vi "Timing FGV.vi"(5 "Time Target (s)":i32=4, 7 "Timer Mode":T1(ring), 8 "Error In":errorcluster) -> (0 "Error Out":errorcluster, 2 "Elapsed Time (s.ms)":dbl format="%#.2f", 3 "Has Time Elapsed":bool)   [LabVIEW 2025, in "Config Tool.lvlib"]
doc: "CLD 3 Exercise\nThis VI is used as a timer functional global. \nNote on reading time when in pause. The developer should not call the read time function when in pause; however, a case structure is used to defensively program the read state for this possibility."
uses:
  Config Tool.lvlib
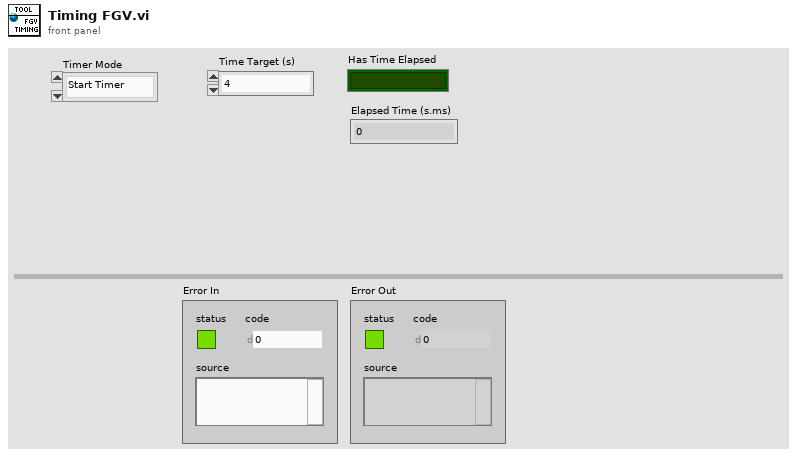
[diagram p1: front panel]
types:
  T1 = enum16{"Start Timer", "Read Time", "Pause", "Resume"}
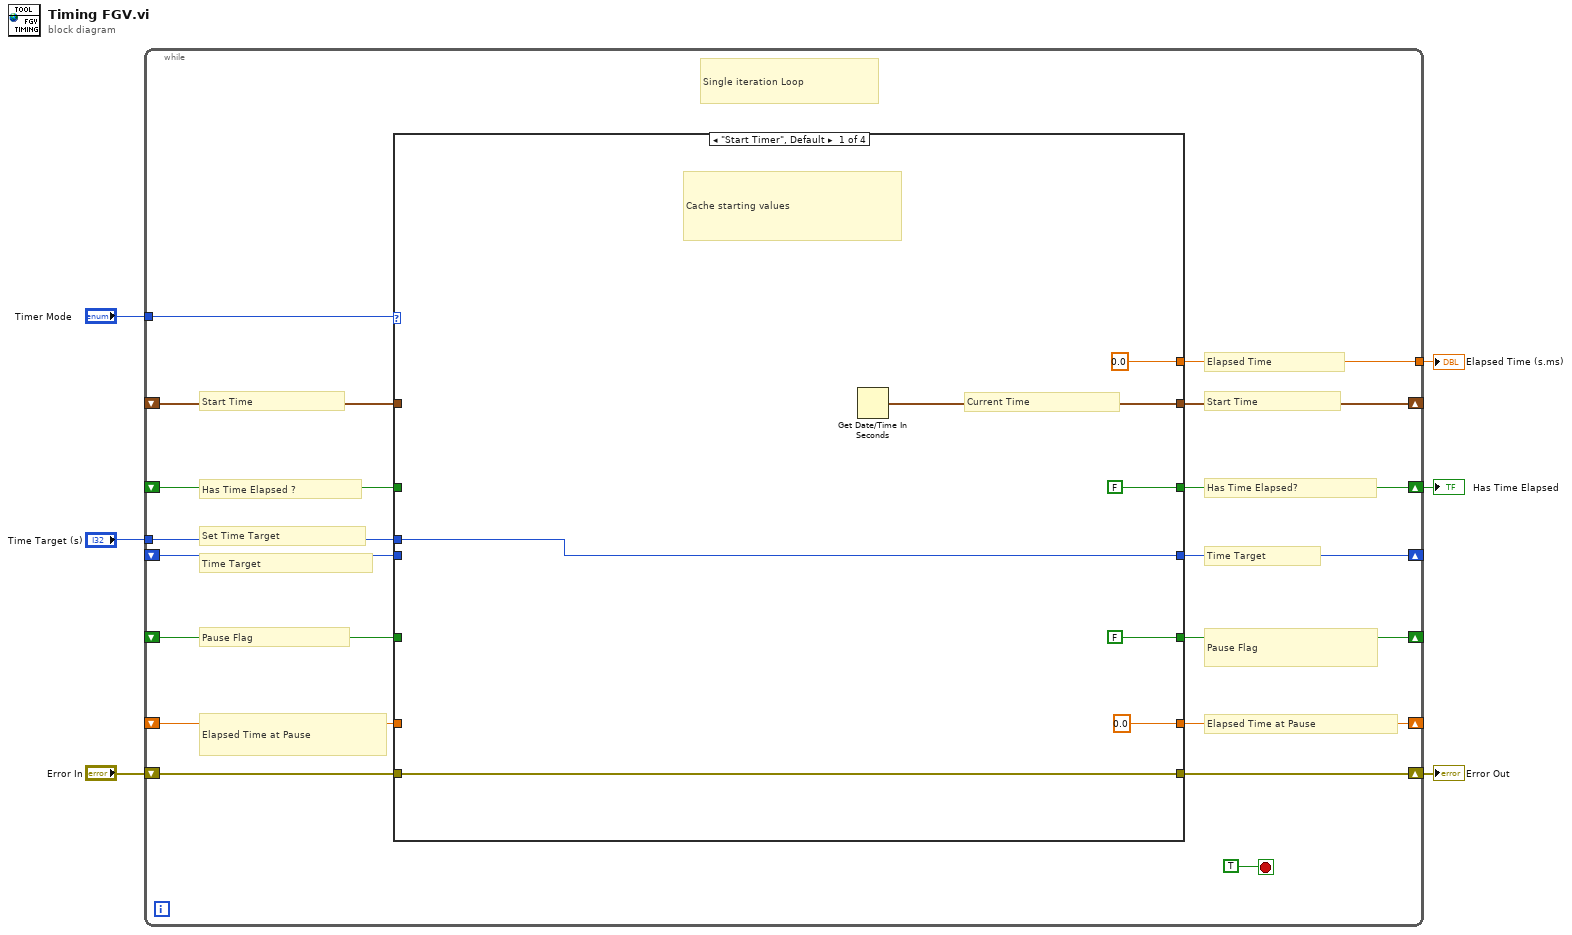
[diagram p0: block diagram]
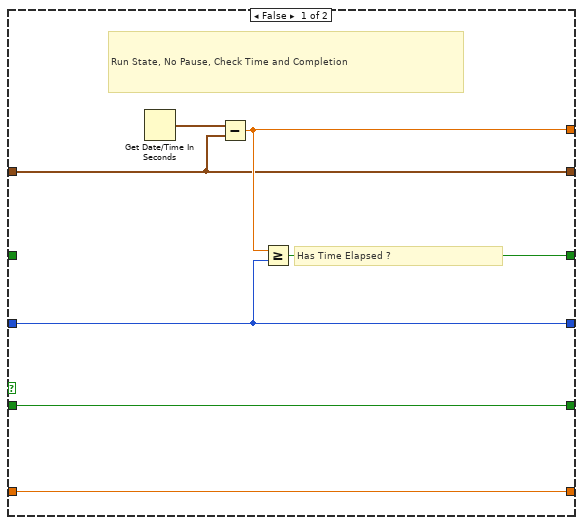
[diagram p3: hidden frame]
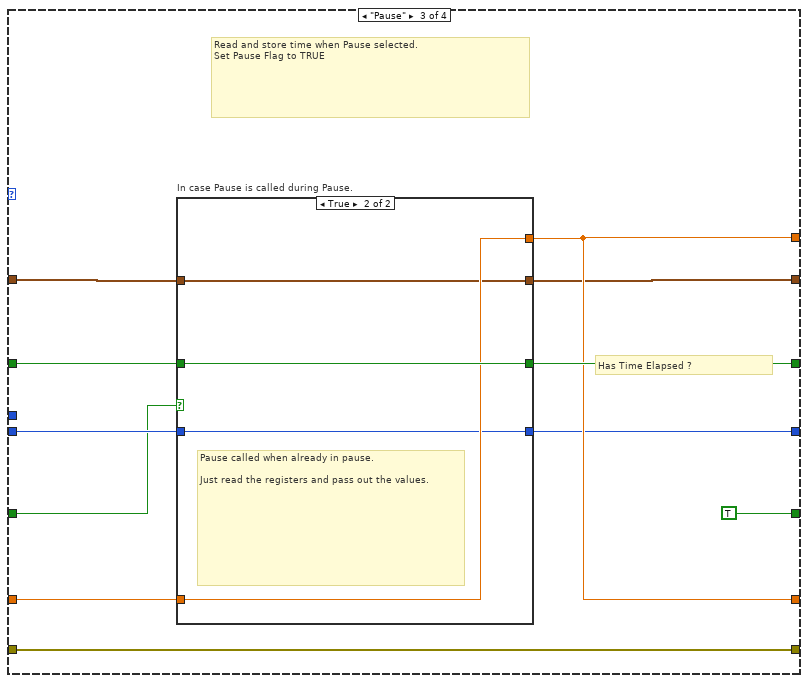
[diagram p4: hidden frame]
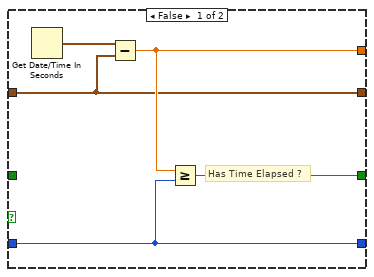
[diagram p5: hidden frame]
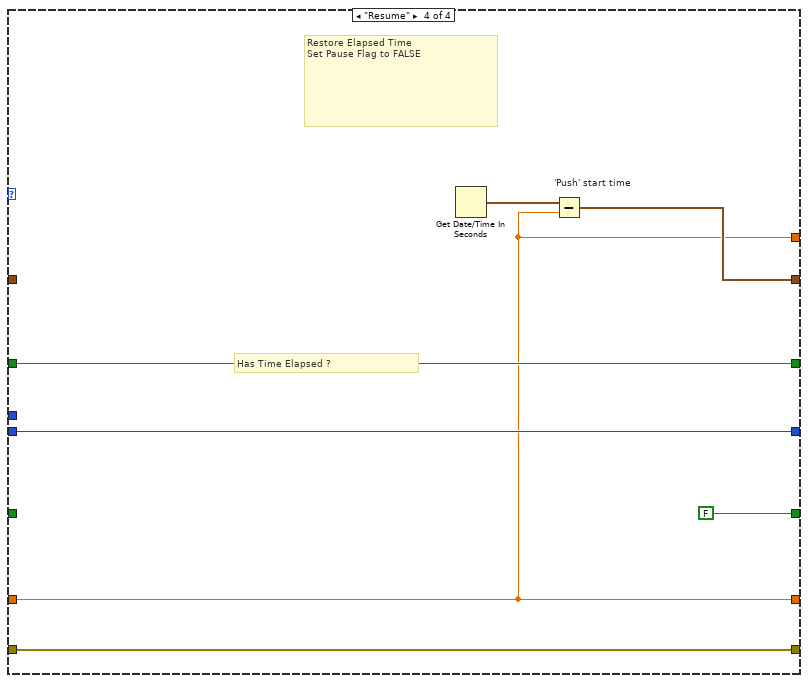
[diagram p6: hidden frame]
diagram:
  n1 = while {
    tunnel: "Timer Mode" -> [w22]
    shift-right: [w20] -> _
    shift-left: _ -> [w19]
    tunnel: [w18] -> w1
    shift-right: [w17] -> w5
    shift-left: "Error In" -> [w16]
    tunnel: "Time Target (s)" -> [w13]
    shift-right: [w14] -> _
    shift-left: _ -> [w15]
    shift-right: [w12] -> w2
    shift-left: _ -> [w11]
    shift-right: [w10] -> _
    shift-left: _ -> [w9]
    shift-right: [w8] -> _
    shift-left: _ -> [w7]
    stop <- TRUE ("stop") stop-if-true
    # "Start Time"
    # "Start Time"
    # "Elapsed Time"
    # "Time Target"
    # "Time Target"
    # "Set Time Target"
    # "Has Time Elapsed?"
    # "Has Time Elapsed ?"
    # "Pause Flag"
    # "Pause Flag"
    # "Elapsed Time at Pause"
    # "Elapsed Time at Pause"
    # "Single iteration Loop"
    n2 = case shown="\"Start Timer\", Default" w22 {
      tunnel: [w29 w33 w53 w74] -> w20
      tunnel: w19 -> [_ w40 w63 _]
      tunnel: [0.0 ("Elapsed Time") w36 w58 w73] -> w18
      tunnel: [w27 w39 w62 w79] -> w17
      tunnel: w16 -> [w27 w39 w62 w79]
      tunnel: w15 -> [_ w38 w61 w78]
      tunnel: [w26 w38 w54 w78] -> w14
      tunnel: w13 -> [w26 _ _ _]
      tunnel: [FALSE w37 w60 w76] -> w12
      tunnel: w11 -> [_ w30 w57 w76]
      tunnel: [FALSE w32 TRUE FALSE] -> w10
      tunnel: w9 -> [_ w31 w56 _]
      tunnel: [0.0 w34 w58 w73] -> w8
      tunnel: w7 -> [_ w35 w55 w73]
      frame "Start Timer", Default {
        # "Current Time"
        # "Cache starting values"
        n3 = Get Date/Time In Seconds() -> (seconds since 1Jan1904=w29:timestamp)
      }
      frame "Read Time" {
        # "Has Time Elapsed ?"
        # "Return Elapsed Time and determine if Time Target has been met."
        n4 = case "In case \"Read Time\" called during Pause (True case)" shown="True" w31 {
          tunnel: w40 -> [w44 w52]
          tunnel: w38 -> [w43 w51]
          tunnel: [w46 w49] -> w37
          tunnel: [w45 w48] -> w36
          tunnel: w35 -> [w41 w48]
          tunnel: [w41 w48] -> w34
          tunnel: [w44 w52] -> w33
          tunnel: [w43 w51] -> _
          tunnel: [w42 w50] -> w32
          tunnel: w31 -> [w42 w50]
          tunnel: w30 -> [_ w49]
          frame False {
            # "Has Time Elapsed ?"
            # "Run State, No Pause, Check Time and Completion"
            n5 = Get Date/Time In Seconds() -> (seconds since 1Jan1904=w47:timestamp)
            n6 = Subtract(x=w47, y=w44) -> (x-y=w45:dbl)
            n7 = Greater Or Equal?(x=w45, y=w43) -> (x >= y?=w46:bool)
          }
          frame True {
            # "Pause State, Just return Shift Registers. Do not call 'Read Time'  when in pause."
          }
        }
      }
      frame "Pause" {
        # "Has Time Elapsed ?"
        # "Read and store time when Pause selected.\nSet Pause Flag to TRUE"
        n8 = case "In case Pause is called during Pause." shown="True" w56 {
          tunnel: w63 -> [w64 w69]
          tunnel: w61 -> [w65 w70]
          tunnel: [w67 w72] -> w60
          tunnel: [w66 w71] -> w58
          tunnel: w57 -> [_ w72]
          tunnel: w55 -> [_ w71]
          tunnel: [w65 w70] -> w54
          tunnel: [w64 w69] -> w53
          frame False {
            # "Has Time Elapsed ?"
            n9 = Get Date/Time In Seconds() -> (seconds since 1Jan1904=w68:timestamp)
            n10 = Subtract(x=w68, y=w64) -> (x-y=w66:dbl)
            n11 = Greater Or Equal?(x=w66, y=w65) -> (x >= y?=w67:bool)
          }
          frame True {
            # "Pause called when already in pause.\n\nJust read the registers and pass out the values."
          }
        }
      }
      frame "Resume" {
        # "Has Time Elapsed ?"
        # "Restore Elapsed Time\nSet Pause Flag to FALSE"
        n12 = Get Date/Time In Seconds() -> (seconds since 1Jan1904=w75:timestamp)
        n13 = Subtract "'Push' start time"(x=w75, y=w73) -> (x-y=w74:timestamp)
      }
    }
  }
  "Error Out" <- w5
  "Has Time Elapsed" <- w2
  "Elapsed Time (s.ms)" <- w1
